vi "글로벌변수.vi"() -> ()   [LabVIEW 2010]
panel:
  in  "while 정지":bool
  out "난수":dbl(graph)
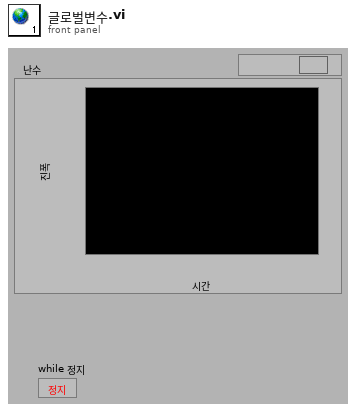
[diagram p1: front panel]
diagram:
